vi "FILE_SAVE.vi"() -> ()   [LabVIEW 2020]
panel:
  out "error out":errorcluster
  in  "File_name":path=path "saved_data"
  in  "Save data":bool
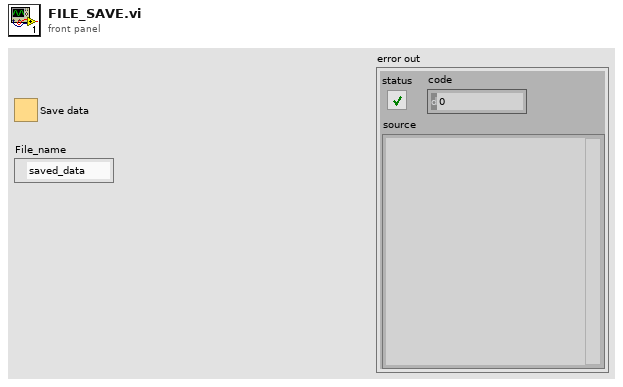
[diagram p1: front panel]
types:
  T1 = enum16{"open", "replace", "create", "open or create", "replace or create", "replace or create with confirmation"}
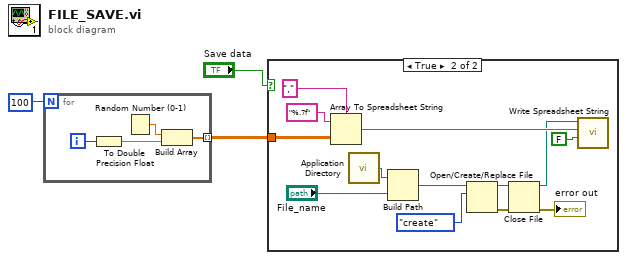
[diagram p0: block diagram]
diagram:
  n1 = for {
    N: 100 -> [_]
    tunnel: [w4] -> w1 mode=indexing
    i -> [w5]
    n2 = To Double Precision Float(number=w5) -> (double precision float=w6:dbl)
    n3 = Random Number (0-1)() -> (number: 0 to 1=w7:dbl)
    n4 = Build Array(w7, w6) -> (w4:dbl[])
  }
  n5 = case shown="True" "Save data" {
    tunnel: w1 -> [_ w11]
    frame False {
    }
    frame True {
      n6 = Array To Spreadsheet String(delimiter (Tab)=",", array=w11, 3:"%.7f" ("format string")) -> (spreadsheet string=w19:string)
      n7 = call <vilib>:"Application Directory.vi"() -> ("Application Directory"=w16:path)
      n8 = Build Path(base path=w16, name or relative path="File_name") -> (appended path=w14:path)
      n9 = Open/Create/Replace File(file path (use dialog)=w14, operation (0:open)=T1."create") -> (refnum out=w17:refnum<file>, error out=w9:errorcluster)  [unwired: 4 in, 1 out]
      n10 = Close File(refnum=w17, error in=w9) -> (path=w13:path, error out=→"error out":errorcluster)
      n11 = call <vilib>:"Write Spreadsheet String.vi"("append to file? (new file:F)"=FALSE, "spreadsheet string"=w19, "file path (dialog if empty)"=w13) -> ()  [unwired: 7 in, 2 out]
    }
  }
